vi "NI VeriStand - Get FIFO Depth.vi"(8 "error in (no error)":errorcluster, 11 "Device Ref in":T1 format="%.0x") -> (0 "error out":errorcluster, 1 "Size FIFO Sink":u32, 2 "Size FIFO Source":u32, 3 "Device Ref out":T1 format="%.0x")   [LabVIEW 2026, in "Custom Devices Storage.lvlib"]
uses:
  Custom Devices Storage.lvlib
  <vilib>/NI VeriStand/Custom Device API/Custom Device Item Ref.ctl
  C:/Users/Administrator/Desktop/Jatin/All DNC DLLs/NationalInstruments.VeriStand.SystemDefinitionAPI.dll
  Jatin/All DNC DLLs/NationalInstruments.VeriStand.SystemDefinitionAPI.dll
  <vilib>/NI VeriStand/Custom Device API/Custom Device API.lvlib
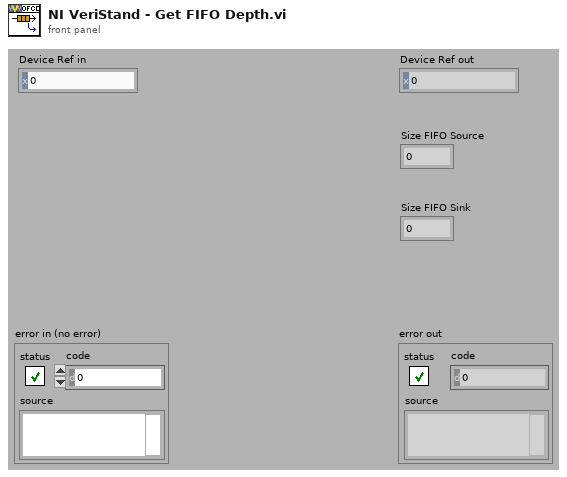
[diagram p1: front panel]
types:
  T1 = typedef "Custom Device API.lvlib/Custom Device Item Ref.ctl" = u64
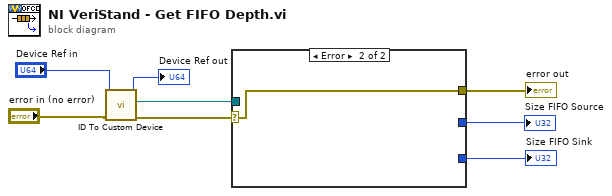
[diagram p0: block diagram]
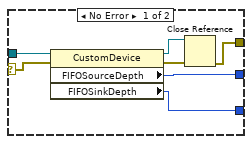
[diagram p2: hidden frame]
diagram:
  n1 = call "ID To Custom Device.vi"("error in (no error)"="error in (no error)", "ID in"="Device Ref in") -> ("error out"=w5:errorcluster, "NationalInstruments.VeriStand.SystemDefinitionAPI.CustomDevice"=w4:refnum<k39>, "ID out"=→"Device Ref out":u64)  [unwired: 7 in]
  n2 = case shown="Error" w5 {
    selector: w5 -> [w14 w16]
    tunnel: w4 -> [w15 _]
    tunnel: [w13 _] -> w3
    tunnel: [w12 _] -> w2
    tunnel: [w9 w16] -> w1
    frame No Error {
      n3 = property class="CustomDevice"(reference=w15, error in=w14) -> (reference out=w10:refnum<k39>, error out=w11:errorcluster, "FIFOSourceDepth"=w13:u32, "FIFOSinkDepth"=w12:u32)
      n4 = Close Reference(reference=w10, error in (no error)=w11) -> (error out=w9:errorcluster)
    }
    frame Error {
    }
  }
  "error out" <- w1
  "Size FIFO Source" <- w3
  "Size FIFO Sink" <- w2
